vi "power.vi"(0 "Channel":T4(ring), 9 "Clear PDP Sticky Faults":bool, 11 "Reset PDP Energy":bool) -> (4 "roboRIO":T3, 6 "Rail Voltages":T2, 8 "PCM":T5, 10 "PDP":T1, 13 "Channel Content":string)   [LabVIEW 2015]
uses:
  Type Defs/power data.ctl
  <vilib>/Rock Robotics/Network Tables/NT Read Number.vi
  <vilib>/Rock Robotics/Network Tables/NT Read Boolean.vi
  <vilib>/Rock Robotics/Network Tables/NT Write Boolean.vi
  <vilib>/Rock Robotics/Network Tables/NT Read String.vi
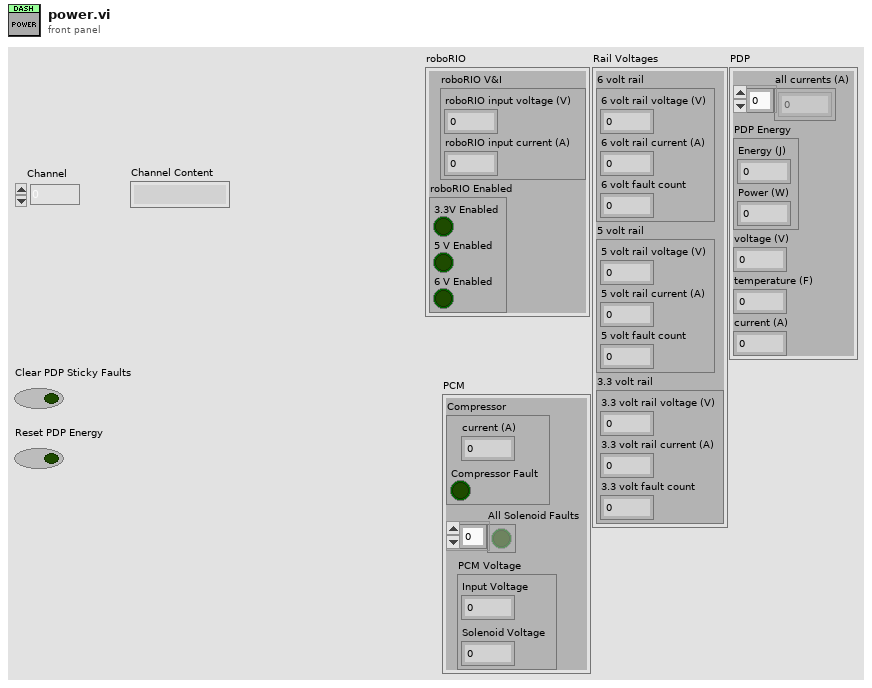
[diagram p1: front panel]
types:
  T1 = cluster{"all currents (A)":dbl[], "PDP Energy":cluster{"Energy (J)":dbl, "Power (W)":dbl}, "voltage (V)":dbl, "temperature (F)":dbl, "current (A)":dbl}
  T2 = cluster{"6 volt rail":cluster{"6 volt rail voltage (V)":dbl, "6 volt rail current (A)":dbl, "6 volt fault count":dbl}, "5 volt rail":cluster{"5 volt rail voltage (V)":dbl, "5 volt rail current (A)":dbl, "5 volt fault count":dbl}, "3.3 volt rail":cluster{"3.3 volt rail voltage (V)":dbl, "3.3 volt rail current (A)":dbl, "3.3 volt fault count":dbl}}
  T3 = cluster{"roboRIO V&I":cluster{"roboRIO input voltage (V)":dbl, "roboRIO input current (A)":dbl}, "roboRIO Enabled":cluster{"3.3V Enabled":bool, "5 V Enabled":bool, "6 V Enabled":bool}}
  T4 = enum16{"0", "1", "2", "3", "4", "5", "6", "7", "8", "9", "10", "11", "12", "13", "14", "15"}
  T5 = cluster{"Compressor":cluster{"current (A)":dbl, "Compressor Fault":bool}, "All Solenoid Faults":bool[], "PCM Voltage":cluster{"Input Voltage":dbl, "Solenoid Voltage":dbl}}
  T6 = cluster{"3.3V Enabled":bool, "5 V Enabled":bool, "6 V Enabled":bool}
  T7 = cluster{"roboRIO V&I":cluster{"roboRIO input voltage (V)":dbl, "roboRIO input current (A)":dbl}, "roboRIO Faults":cluster{"3.3V User Rail Short":bool, "5 V User Rail Short":bool, "6 V User Rail Short":bool}}
  T8 = cluster{"all currents (A)":dbl[], "PDP Energy":cluster{"Energy (J)":dbl, "Power (W)":dbl}, "voltage (V)":dbl, "Temperature (F)":dbl, "Current (A)":dbl}
  T9 = typedef "power data.ctl" = cluster{"roboRIO":cluster{"roboRIO V&I":cluster{"roboRIO input voltage (V)":dbl, "roboRIO input current (A)":dbl}, "roboRIO Enabled":cluster{"3.3V Enabled":bool, "5 V Enabled":bool, "6 V Enabled":bool}}, "Rail Voltages":cluster{"6 volt rail":cluster{"6 volt rail voltage (V)":dbl, "6 volt rail current (A)":dbl, "6 volt fault count":dbl}, "5 volt rail":cluster{"5 volt rail voltage (V)":dbl, "5 volt rail current (A)":dbl, "5 volt fault count":dbl}, "3.3 volt rail":cluster{"3.3 volt rail voltage (V)":dbl, "3.3 volt rail current (A)":dbl, "3.3 volt fault count":dbl}}, "PDP":cluster{"all currents (A)":dbl[], "PDP Energy":cluster{"Energy (J)":dbl, "Power (W)":dbl}, "voltage (V)":dbl, "temperature (F)":dbl, "current (A)":dbl}}
  T10 = cluster{"6 volt rail":cluster{"6 volt rail voltage (V)":dbl, "6 volt rail current (A)":dbl, "6 volt rail fault count":dbl}, "5 volt rail":cluster{"5 volt rail voltage (V)":dbl, "5 volt rail current (A)":dbl, "5 volt rail fault count":dbl}, "3.3 volt rail":cluster{"3.3 volt rail voltage (V)":dbl, "3.3 volt rail current (A)":dbl, "3.3 volt rail fault count":dbl}}
  T11 = cluster{"3.3 volt rail voltage (V)":dbl, "3.3 volt rail current (A)":dbl, "3.3 volt rail fault count":dbl}
  T12 = cluster{"5 volt rail voltage (V)":dbl, "5 volt rail current (A)":dbl, "5 volt rail fault count":dbl}
  T13 = cluster{"6 volt rail voltage (V)":dbl, "6 volt rail current (A)":dbl, "6 volt rail fault count":dbl}
  T14 = cluster{"roboRIO input voltage (V)":dbl, "roboRIO input current (A)":dbl}
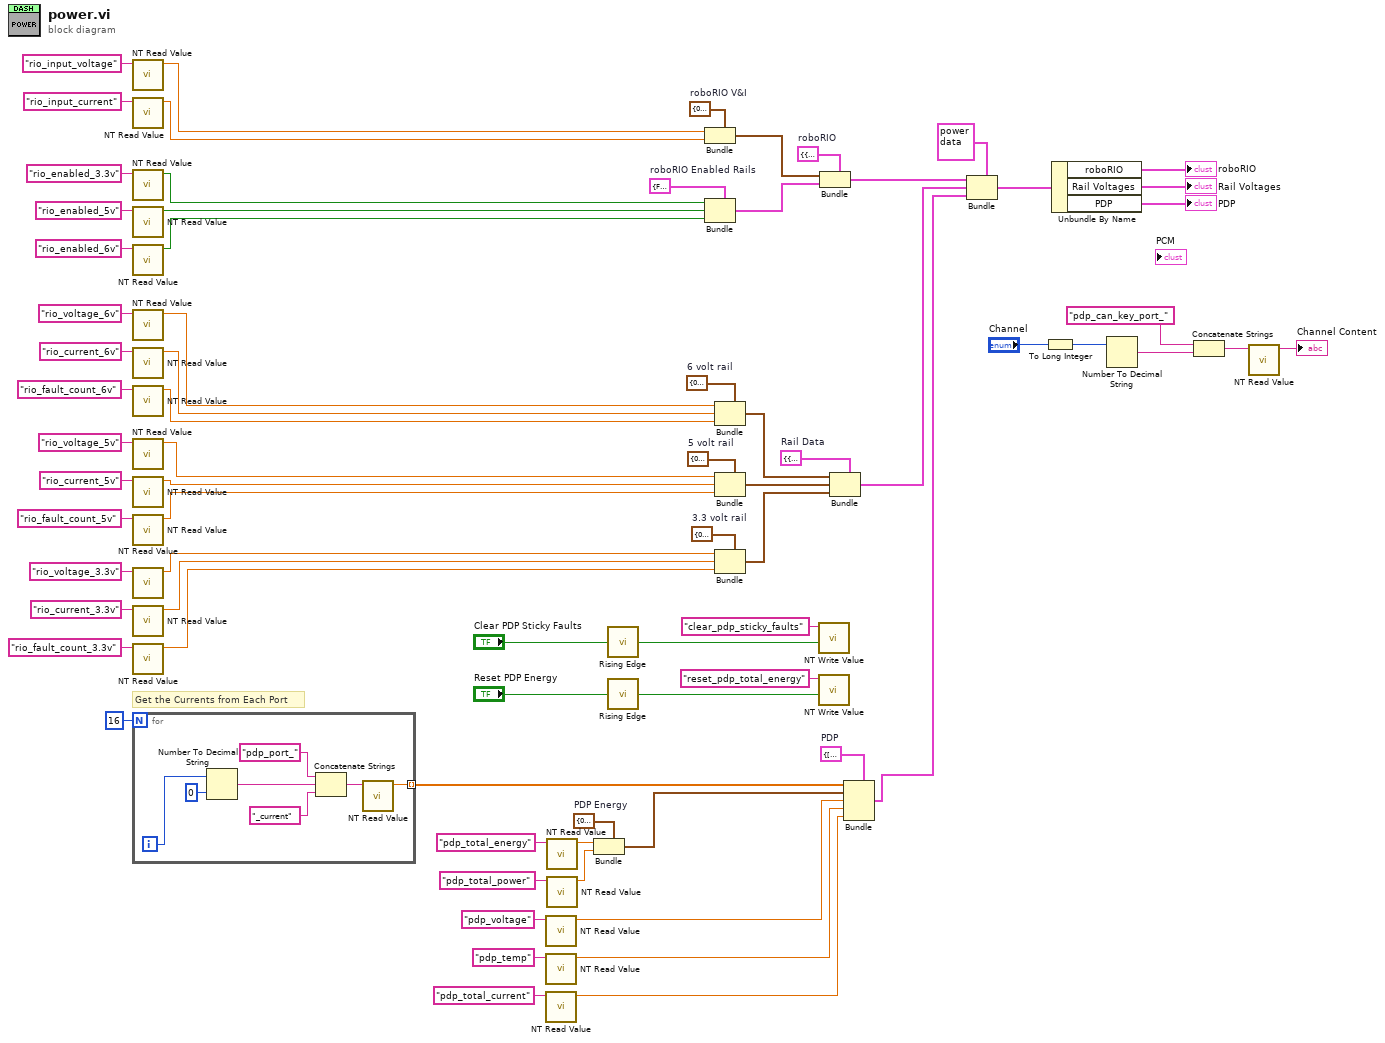
[diagram p0: block diagram]
diagram:
  w68 = T6 {"3.3V Enabled"=FALSE, "5 V Enabled"=FALSE, "6 V Enabled"=FALSE}  # roboRIO Enabled Rails
  w69 = T7 {"roboRIO V&I"={"roboRIO input voltage (V)"=0.0, "roboRIO input current (A)"=0.0}, "roboRIO Faults"={"3.3V User Rail Short"=FALSE, "5 V User Rail Short"=FALSE, "6 V User Rail Short"=FALSE}}  # roboRIO
  w58 = cluster{"Energy (J)":dbl, "Power (W)":dbl} {"Energy (J)"=0.0, "Power (W)"=0.0}  # PDP Energy
  w57 = T8 {"all currents (A)"=[], "PDP Energy"={"Energy (J)"=0.0, "Power (W)"=0.0}, "voltage (V)"=0.0, "Temperature (F)"=0.0, "Current (A)"=0.0}  # PDP
  w63 = T10 {"6 volt rail"={"6 volt rail voltage (V)"=0.0, "6 volt rail current (A)"=0.0, "6 volt rail fault count"=0.0}, "5 volt rail"={"5 volt rail voltage (V)"=0.0, "5 volt rail current (A)"=0.0, "5 volt rail fault count"=0.0}, "3.3 volt rail"={"3.3 volt rail voltage (V)"=0.0, "3.3 volt rail current (A)"=0.0, "3.3 volt rail fault count"=0.0}}  # Rail Data
  w60 = T11 {"3.3 volt rail voltage (V)"=0.0, "3.3 volt rail current (A)"=0.0, "3.3 volt rail fault count"=0.0}  # 3.3 volt rail
  w61 = T12 {"5 volt rail voltage (V)"=0.0, "5 volt rail current (A)"=0.0, "5 volt rail fault count"=0.0}  # 5 volt rail
  w62 = T13 {"6 volt rail voltage (V)"=0.0, "6 volt rail current (A)"=0.0, "6 volt rail fault count"=0.0}  # 6 volt rail
  w67 = T14 {"roboRIO input voltage (V)"=0.0, "roboRIO input current (A)"=0.0}  # roboRIO V&I
  # "Get the Currents from Each Port"
  n1 = call-poly <vilib>:"NT Read Value.vi"("Name"="rio_input_voltage") -> ("Numeric"=w54:dbl)  [unwired: 9 in, 1 out]
  n2 = call-poly <vilib>:"NT Read Value.vi"("Name"="rio_input_current") -> ("Numeric"=w53:dbl)  [unwired: 9 in, 1 out]
  n3 = call-poly <vilib>:"NT Read Value.vi"("Name"="rio_enabled_3.3v") -> ("Boolean"=w49:bool)  [unwired: 9 in, 1 out]
  n4 = call-poly <vilib>:"NT Read Value.vi"("Name"="rio_enabled_5v") -> ("Boolean"=w48:bool)  [unwired: 9 in, 1 out]
  n5 = call-poly <vilib>:"NT Read Value.vi"("Name"="rio_enabled_6v") -> ("Boolean"=w47:bool)  [unwired: 9 in, 1 out]
  n6 = call-poly <vilib>:"NT Read Value.vi"("Name"="rio_voltage_6v") -> ("Numeric"=w43:dbl)  [unwired: 9 in, 1 out]
  n7 = call-poly <vilib>:"NT Read Value.vi"("Name"="rio_current_6v") -> ("Numeric"=w41:dbl)  [unwired: 9 in, 1 out]
  n8 = call-poly <vilib>:"NT Read Value.vi"("Name"="rio_fault_count_6v") -> ("Numeric"=w42:dbl)  [unwired: 9 in, 1 out]
  n9 = call-poly <vilib>:"NT Read Value.vi"("Name"="rio_voltage_5v") -> ("Numeric"=w34:dbl)  [unwired: 9 in, 1 out]
  n10 = call-poly <vilib>:"NT Read Value.vi"("Name"="rio_current_5v") -> ("Numeric"=w33:dbl)  [unwired: 9 in, 1 out]
  n11 = call-poly <vilib>:"NT Read Value.vi"("Name"="rio_fault_count_5v") -> ("Numeric"=w32:dbl)  [unwired: 9 in, 1 out]
  n12 = call-poly <vilib>:"NT Read Value.vi"("Name"="rio_voltage_3.3v") -> ("Numeric"=w31:dbl)  [unwired: 9 in, 1 out]
  n13 = call-poly <vilib>:"NT Read Value.vi"("Name"="rio_current_3.3v") -> ("Numeric"=w30:dbl)  [unwired: 9 in, 1 out]
  n14 = call-poly <vilib>:"NT Read Value.vi"("Name"="rio_fault_count_3.3v") -> ("Numeric"=w29:dbl)  [unwired: 9 in, 1 out]
  n15 = for {
    N: 16 -> [_]
    tunnel: [w76] -> w27 mode=indexing
    i -> [w80]
    n16 = Number To Decimal String(number=w80, width (-)=i16 0) -> (decimal integer string=w78:string)
    n17 = Concatenate Strings("pdp_port_" ("Name"), w78, "_current" ("Name")) -> (w77:string)
    n18 = call-poly <vilib>:"NT Read Value.vi"("Name"=w77) -> ("Numeric"=w76:dbl)  [unwired: 9 in, 1 out]
  }
  n19 = call-poly <vilib>:"NT Read Value.vi"("Name"="pdp_voltage") -> ("Numeric"=w18:dbl)  [unwired: 9 in, 1 out]
  n20 = call-poly <vilib>:"NT Read Value.vi"("Name"="pdp_temp") -> ("Numeric"=w17:dbl)  [unwired: 9 in, 1 out]
  n21 = call-poly <vilib>:"NT Read Value.vi"("Name"="pdp_total_current") -> ("Numeric"=w16:dbl)  [unwired: 9 in, 1 out]
  n22 = call-poly <vilib>:"NT Read Value.vi"("Name"="pdp_total_energy") -> ("Numeric"=w24:dbl)  [unwired: 9 in, 1 out]
  n23 = call-poly <vilib>:"NT Read Value.vi"("Name"="pdp_total_power") -> ("Numeric"=w23:dbl)  [unwired: 9 in, 1 out]
  n24 = Bundle(cluster=w58, "Energy (J)"=w24, "Power (W)"=w23) -> (w22:cluster{"Energy (J)":dbl, "Power (W)":dbl})
  n25 = call "Rising Edge.vi"("Input"="Clear PDP Sticky Faults") -> ("Rising Edge"=w15:bool)
  n26 = call "Rising Edge.vi"("Input"="Reset PDP Energy") -> ("Rising Edge"=w12:bool)
  n27 = Bundle(cluster=w67, "roboRIO input voltage (V)"=w54, "roboRIO input current (A)"=w53) -> (w70:T14)
  n28 = Bundle(cluster=w68, "3.3V Enabled"=w49, "5 V Enabled"=w48, "6 V Enabled"=w47) -> (w71:T6)
  n29 = Bundle(cluster=w62, "6 volt rail voltage (V)"=w43, "6 volt rail current (A)"=w41, "6 volt rail fault count"=w42) -> (w64:T13)
  n30 = Bundle(cluster=w61, "5 volt rail voltage (V)"=w34, "5 volt rail current (A)"=w33, "5 volt rail fault count"=w32) -> (w65:T12)
  n31 = Bundle(cluster=w60, "3.3 volt rail voltage (V)"=w31, "3.3 volt rail current (A)"=w30, "3.3 volt rail fault count"=w29) -> (w66:T11)
  n32 = call-poly <vilib>:"NT Write Value.vi"("Boolean"=w15, "Name"="clear_pdp_sticky_faults") -> ()  [unwired: 9 in, 1 out]
  n33 = call-poly <vilib>:"NT Write Value.vi"("Boolean"=w12, "Name"="reset_pdp_total_energy") -> ()  [unwired: 9 in, 1 out]
  n34 = Bundle(cluster=w69, "roboRIO V&I"=w70, "roboRIO Faults"=w71) -> (w11:T7)
  n35 = Bundle(cluster=w63, "6 volt rail"=w64, "5 volt rail"=w65, "3.3 volt rail"=w66) -> (w10:T10)
  n36 = Bundle(cluster=w57, "all currents (A)"=w27, "PDP Energy"=w22, "voltage (V)"=w18, "Temperature (F)"=w17, "Current (A)"=w16) -> (w9:T8)
  n37 = Bundle(cluster=T9 {"roboRIO"={"roboRIO V&I"={"roboRIO input voltage (V)"=0.0, "roboRIO input current (A)"=0.0}, "roboRIO Enabled"={"3.3V Enabled"=FALSE, "5 V Enabled"=FALSE, "6 V Enabled"=FALSE}}, "Rail Voltages"={"6 volt rail"={"6 volt rail voltage (V)"=0.0, "6 volt rail current (A)"=0.0, "6 volt fault count"=0.0}, "5 volt rail"={"5 volt rail voltage (V)"=0.0, "5 volt rail current (A)"=0.0, "5 volt fault count"=0.0}, "3.3 volt rail"={"3.3 volt rail voltage (V)"=0.0, "3.3 volt rail current (A)"=0.0, "3.3 volt fault count"=0.0}}, "PDP"={"all currents (A)"=[], "PDP Energy"={"Energy (J)"=0.0, "Power (W)"=0.0}, "voltage (V)"=0.0, "temperature (F)"=0.0, "current (A)"=0.0}} ("Power Data"), "roboRIO"=w11, "Rail Voltages"=w10, "PDP"=w9) -> (w75:T9)
  n38 = To Long Integer(number="Channel") -> (32bit integer=w5:i32)
  n39 = Unbundle By Name(w75) -> ("roboRIO"=→"roboRIO":T3, "Rail Voltages"=→"Rail Voltages":T2, "PDP"=→"PDP":T1)
  n40 = Number To Decimal String(number=w5) -> (decimal integer string=w4:string)  [unwired: 1 in]
  n41 = Concatenate Strings("pdp_can_key_port_" ("string"), w4) -> (w2:string)
  n42 = call-poly <vilib>:"NT Read Value.vi"("Name"=w2) -> ("String"=→"Channel Content":string)  [unwired: 9 in, 1 out]
